vi "Drive.vi"(8 "error in":errorcluster) -> (0 "error out":errorcluster)   [LabVIEW 2016]
uses:
  Sprocket/src/Refname/Queues.ctl
  Sprocket/src/Refname/Actuators.ctl
  Drive States.ctl
  Sprocket/src/Action/Action Name.ctl
  Sprocket/src/Refname/Refname to String (Queue).vi
  <vilib>/addons/control/pid/pid.llb/PID (DBL).vi
  Main/Robot Global Data.vi
  Sprocket/lib/Sprocket.lvlib
  <vilib>/addons/control/pid/NI_PID_pid.lvlib
panel:
  in  "PID gains":T1={"proportional gain (Kc)"=0.025, "integral time (Ti, min)"=0.0, "derivative time (Td, min)"=0.0} {"derivative time (Td, min)" format="%.3f"; "integral time (Ti, min)" format="%.3f"; "proportional gain (Kc)" format="%.3f"}
  in  "output range":cluster{"output high":dbl, "output low":dbl}={"output high"=0.6, "output low"=-0.6} {"output low" format="%.2f"; "output high" format="%.2f"}
  # "Auto Rotate PID"
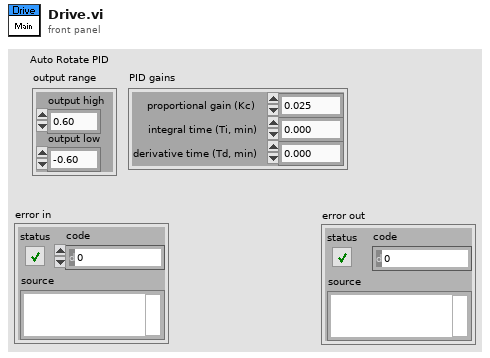
[diagram p1: front panel]
types:
  T1 = cluster{"proportional gain (Kc)":dbl, "integral time (Ti, min)":dbl, "derivative time (Td, min)":dbl}
  T2 = typedef "Sprocket.lvlib/Actuators.ctl" = enum16{"Drive Motor 1 (R)", "Drive Motor 2 (R)", "Drive Motor 3 (R)", "Drive Motor 4 (L)", "Drive Motor 5 (L)", "Drive Motor 6 (L)", "Collector Motor", "Collector Solenoid", "Compressor", "SonicShifter", "Gyro", "UltraSonic Front Left", "UltraSonic Back Left", "Wedge Motor", "Wedge LS"}
  T3 = typedef "Drive States.ctl" = enum16{"Idle", "Teleop", "Start Rotate", "Do Rotate", "Stop Rotate", "Start Throttle", "Do Throttle", "Stop Throttle"}
  T4 = typedef "Sprocket.lvlib/Queues.ctl" = enum16{"Input", "Drive", "Collector", "Shifter", "Wedge"}
  T5 = typedef "WPI_MotorControlDeviceRef.ctl" = cluster{"DeviceStatus":errorcluster, "Type":T6, "PWM":cluster{"PWM Channel":T7, "DeadBand":T8}, "CAN":cluster{"Device Number":u8, "SetOutput VI Ref":variant, "GetOutput VI Ref":variant, "Enable VI Ref":variant, "Disable VI Ref":variant, "Data":variant}, "Invert":bool}
  T6 = typedef "WPI_MotorControlType.ctl" = enum16{"PWM", "CAN"}
  T7 = typedef "FPGA_DIOPWMChannel.ctl" = enum8{"PWM 0", "PWM 1", "PWM 2", "PWM 3", "PWM 4", "PWM 5", "PWM 6", "PWM 7", "PWM 8", "PWM 9", "PWM MXP 0", "PWM MXP 1", "PWM MXP 2", "PWM MXP 3", "PWM MXP 4", "PWM MXP 5", "PWM MXP 6", "PWM MXP 7", "PWM MXP 8", "PWM MXP 9", "Invalid"}
  T8 = typedef "WPI_PWMDeadband.ctl" = cluster{"Name":string, "maxPositivePwm":i32, "minPositivePwm":i32, "centerPwm":i32, "maxNegativePwm":i32, "minNegativePwm":i32, "angularRange":u16}
  T9 = typedef "WPI_GyroDevRef.ctl" = cluster{"DevStatus":errorcluster, "Analog Channel":T10, "Offset":dbl, "Gain (VoltsPerDegree/Second)":dbl, "Gyro Type":enum16{"Analog", "XRS450"}, "Handle":i32, "SPI Bus":T11, "Device Found":bool, "Sample Rate":dbl, "Calibrate On Open":bool}
  T10 = typedef "FPGA_AIChannel.ctl" = enum8{"AI 0", "AI 1", "AI 2", "AI 3", "AI MXP 0", "AI MXP 1", "AI MXP 2", "AI MXP 3", "Invalid"}
  T11 = typedef "spi_bus.ctl" = enum16{"SPI On-Board, CS0", "SPI On-Board, CS1", "SPI On-Board, CS2", "SPI On-Board, CS3", "SPI MXP", "Invalid"}
  T12 = typedef "Sprocket.lvlib/Action Name.ctl" = enum16{"No Action", "Drive Train Both", "Drive Train Rotate", "Drive Train Throttle", "Collector Motor Roll", "Collector Motor Eject", "Collector Motor Collect", "Collector Motor Stop", "Collector Extend", "Collector Retract", "Shifter High", "Shifter Low", "Collector Motor Stall", "Wedge Roll"}
  T13 = typedef "Sprocket.lvlib/Action.ctl" = cluster{"Name":T12, "Priority":i32, "Data":variant}
  T14 = typedef "WPI_CANTalonSRX_GlobalStatus.ctl" = cluster{"Applied Throttle":dbl, "Module Enabled":bool, "CAN Error":errorcluster, "Closed Loop Error":dbl, "Forward Limit Switch Closed":bool, "Reverse Limit Switch Closed":bool, "Sensor Position":dbl, "Sensor Velocity":dbl, "Current":dbl, "Sticky Fault - Over Temp":bool, "Sticky Fault - Under Voltage":bool, "Sticky Fault - Forward Limit":bool, "Sticky Fault - Reverse Limit":bool, "Sticky Fault - Forward Soft Limit":bool, "Sticky Fault - Reverse Soft Limit":bool, "Brake is Enabled":bool, "Encoder Position":dbl, "Encoder Velocity":dbl, "Encoder Index Count":dbl, "Encoder A Pin State":bool, "Encoder B Pin State":bool, "Encoder Index Pin State":bool, "Analog In":dbl, "Analog In Velocity":dbl, "Temperature (C)":dbl, "Battery Voltage":dbl, "Control 5 Is Supported":bool, "Current Profile Slot Select":dbl, "Pos Div 8":bool, "Vel Div 4":bool, "Pulse Width Position":i32, "Pulse Width Velocity":i32, "Pulse Width Rise To Rise (us)":i32, "Pulse Width Rise To Fall (us)":i32, "Mot Prof Active Is Under Run":bool, "Mot Prof Active Has Under Run":bool, "Mot Prof Active Is Last":bool, "Mot Prof Active Velocity Only":bool, "Mot Prof Active Is Valid":bool, "Mot Prof Buffer Is Full":bool, "Mot Prof Active Profile Slot Select":i32, "Mot Prof NextID":i32, "Mot Prof Count":i32, "Mot Prof Active Velocity":dbl, "Mot Prof Active Position":dbl, "Mot Prof Output Enable":i32}
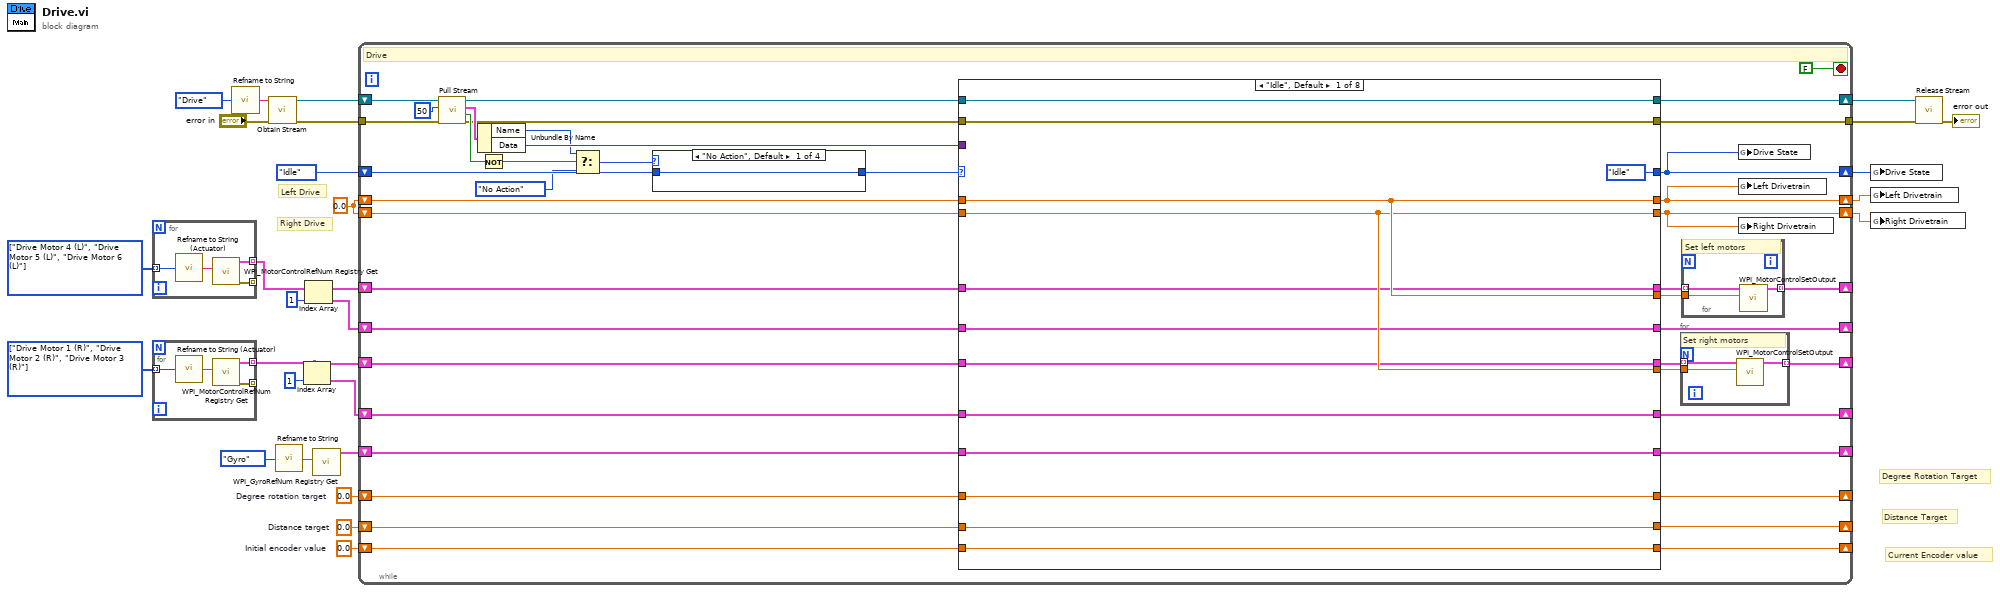
[diagram p0: block diagram]
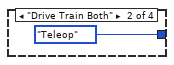
[diagram p2: hidden frame]
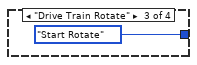
[diagram p3: hidden frame]
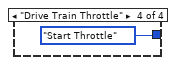
[diagram p4: hidden frame]
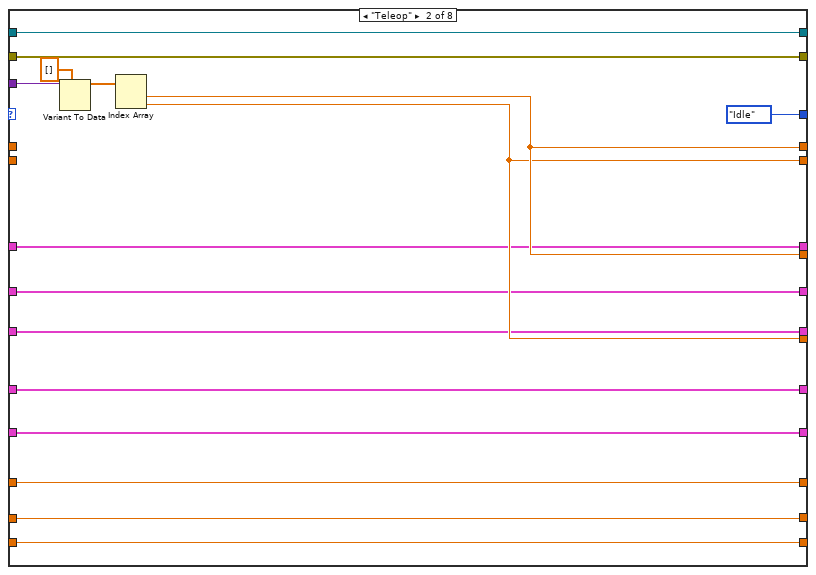
[diagram p5: hidden frame]
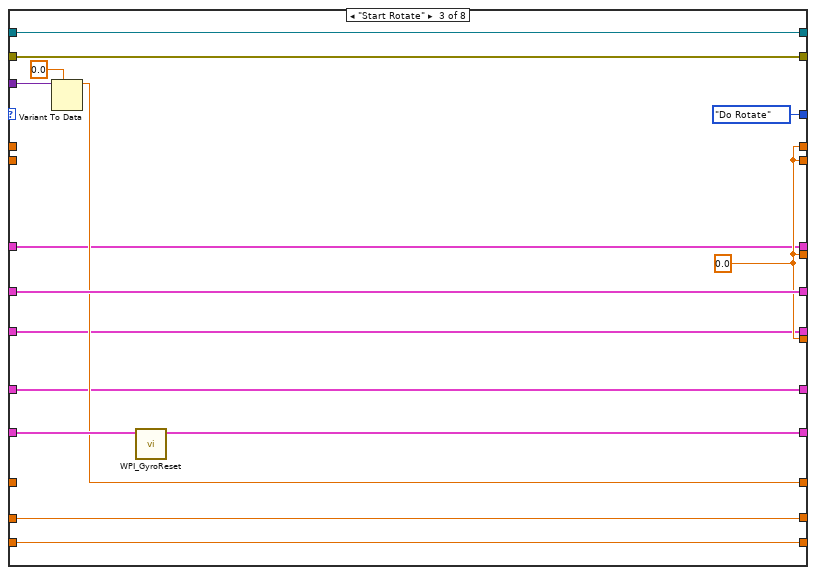
[diagram p6: hidden frame]
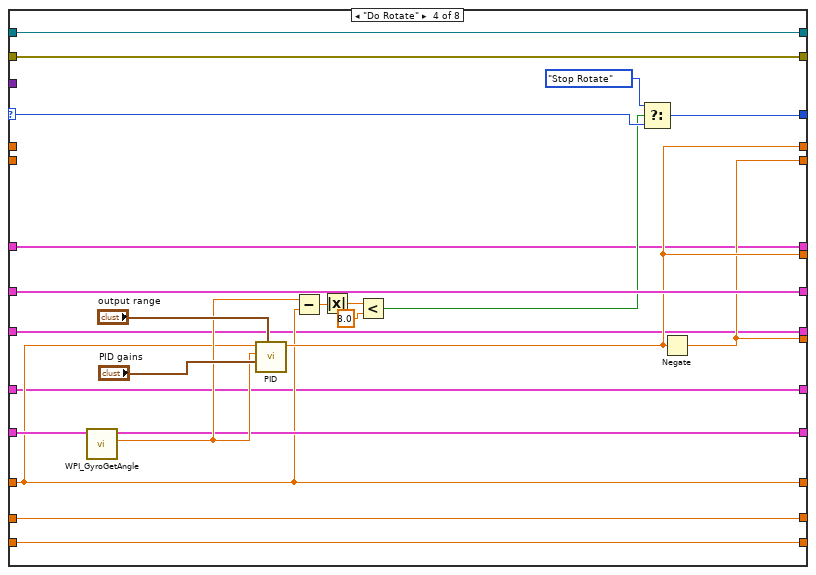
[diagram p7: hidden frame]
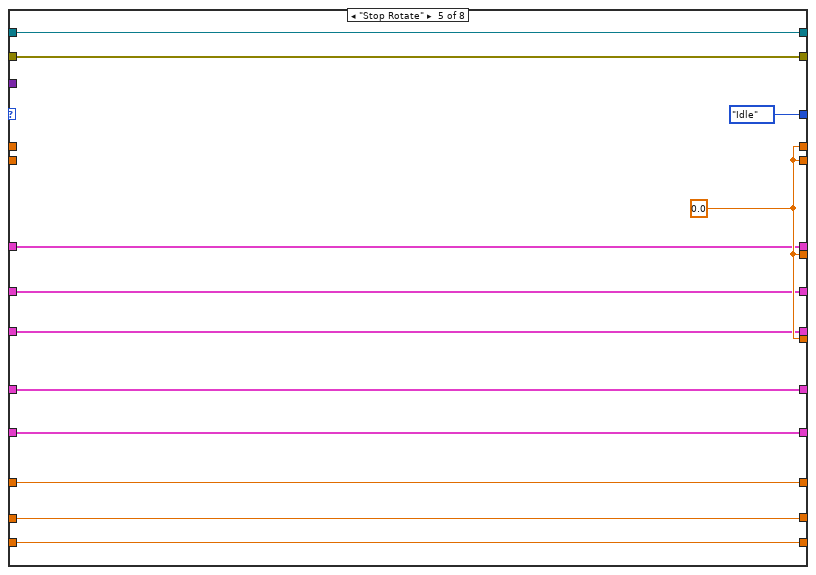
[diagram p8: hidden frame]
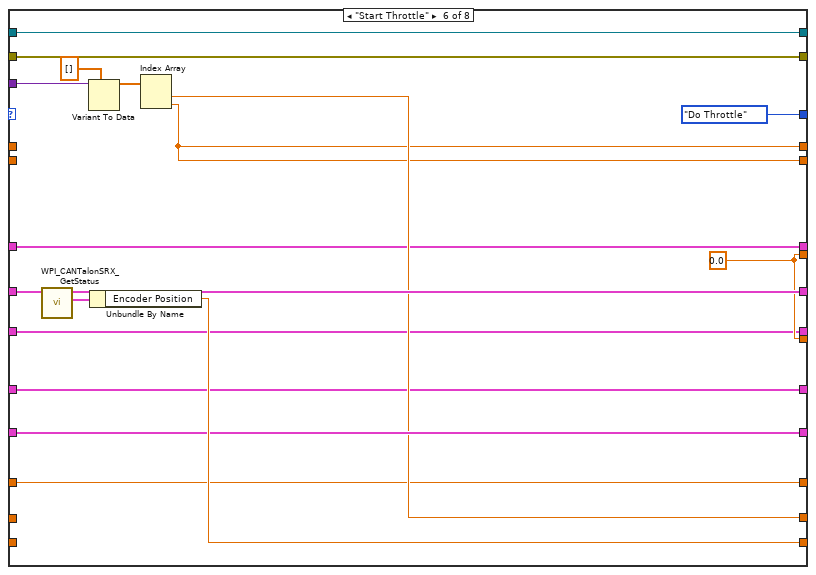
[diagram p9: hidden frame]
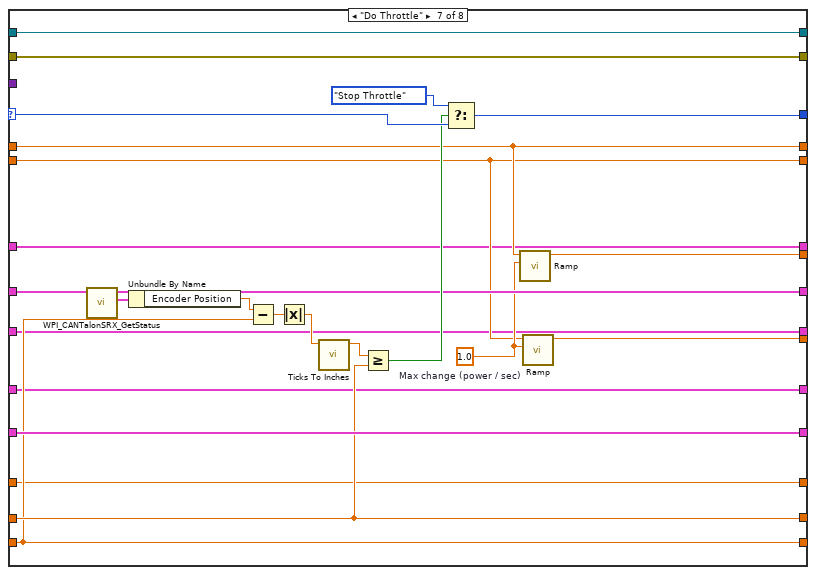
[diagram p10: hidden frame]
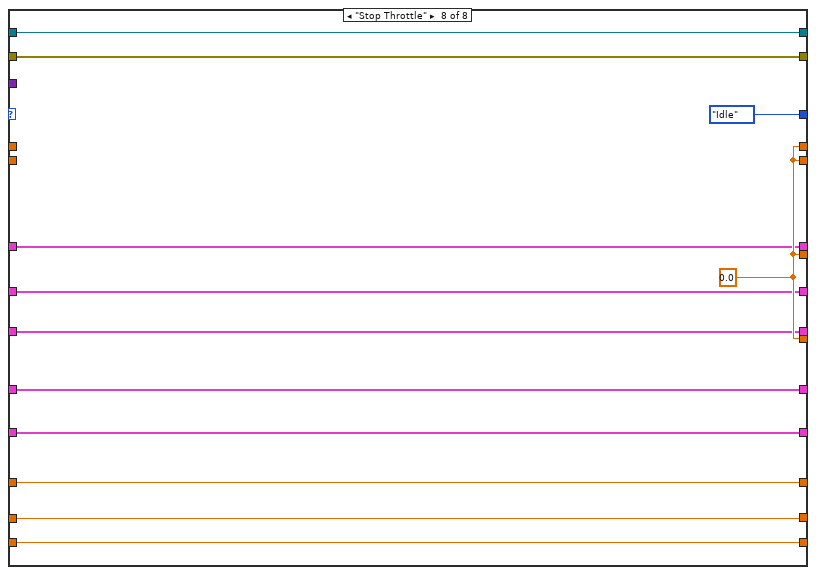
[diagram p11: hidden frame]
diagram:
  w5 = 0.0
  w15 = T2[] [enum."Drive Motor 4 (L)", enum."Drive Motor 5 (L)", enum."Drive Motor 6 (L)"] items=["Drive Motor 1 (R)", "Drive Motor 2 (R)", "Drive Motor 3 (R)", "Drive Motor 4 (L)", "Drive Motor 5 (L)", "Drive Motor 6 (L)", "Collector Motor", "Collector Solenoid", "Compressor", "SonicShifter", "Gyro", "UltraSonic Front Left", "UltraSonic Back Left", "Wedge Motor", "Wedge LS"]
  w17 = T2[] [enum."Drive Motor 1 (R)", enum."Drive Motor 2 (R)", enum."Drive Motor 3 (R)"] items=["Drive Motor 1 (R)", "Drive Motor 2 (R)", "Drive Motor 3 (R)", "Drive Motor 4 (L)", "Drive Motor 5 (L)", "Drive Motor 6 (L)", "Collector Motor", "Collector Solenoid", "Compressor", "SonicShifter", "Gyro", "UltraSonic Front Left", "UltraSonic Back Left", "Wedge Motor", "Wedge LS"]
  w20 = 0.0  # Initial encoder value
  w19 = 0.0  # Distance target
  w18 = 0.0  # Degree rotation target
  # "Right Drive"
  # "Left Drive"
  # "Current Encoder value"
  # "Distance Target"
  # "Degree Rotation Target"
  n1 = for {
    tunnel: w15 -> [w30] mode=indexing
    tunnel: [w29] -> _ mode=indexing
    tunnel: [w28] -> w10 mode=indexing
    n2 = call "Refname to String (Actuator).vi"("Actuator Refname"=w30) -> ("Refnum Name"=w31:string)
    n3 = call <vilib>:"WPI_MotorControlRefNum Registry Get.vi"("refnum name"=w31) -> ("error out"=w29:errorcluster, "MotorControlDevRef"=w28:T5)  [unwired: 9 in]
  }
  n4 = for {
    tunnel: w17 -> [w34] mode=indexing
    tunnel: [w33] -> _ mode=indexing
    tunnel: [w32] -> w1 mode=indexing
    n5 = call "Refname to String (Actuator).vi"("Actuator Refname"=w34) -> ("Refnum Name"=w35:string)
    n6 = call <vilib>:"WPI_MotorControlRefNum Registry Get.vi"("refnum name"=w35) -> ("error out"=w33:errorcluster, "MotorControlDevRef"=w32:T5)  [unwired: 9 in]
  }
  n7 = call-poly "Refname to String.vi"("Queue Refname"=Queues."Drive" ("Refname (Queue)")) -> ("Refnum Name"=w21:string)
  n8 = call "Obtain Stream.vi"("error in (no error)"="error in", "Name"=w21) -> ("error out"=w25:errorcluster, "stream out"=w24:refnum<queue>)  [unwired: 8 in]
  n9 = call-poly "Refname to String.vi"("Actuator Refname"=Actuators."Gyro") -> ("Refnum Name"=w13:string)
  n10 = Index Array(array=w1, index=1) -> (element=w2:T5)
  n11 = Index Array(array=w10, index=1) -> (element=w8:T5)
  n12 = call <vilib>:"WPI_GyroRefNum Registry Get.vi"("refnum name"=w13) -> ("GyroDevRef"=w11:T9)  [unwired: 9 in, 1 out]
  n13 = while {
    shift-right: [w45] -> w27
    shift-left: w24 -> [w72]
    shift-right: [w70] -> w3
    shift-left: w5 -> [w68]
    shift-right: [w71] -> w4
    shift-left: w5 -> [w69]
    tunnel: w25 -> [w73]
    tunnel: [w74] -> w26
    shift-right: [w58] -> _
    shift-left: w10 -> [w40]
    shift-right: [w57] -> _
    shift-left: w1 -> [w38]
    shift-right: [w62] -> _
    shift-left: w18 -> [w61]
    shift-right: [w54] -> _
    shift-left: w19 -> [w56]
    shift-right: [w53] -> _
    shift-left: w20 -> [w55]
    shift-right: [w51] -> w7
    shift-left: Drive_States."Idle" ("Enum") -> [w65]
    shift-right: [w63] -> _
    shift-left: w11 -> [w47]
    shift-right: [w52] -> _
    shift-left: w8 -> [w49]
    shift-right: [w36] -> _
    shift-left: w2 -> [w48]
    stop <- FALSE stop-if-true
    # "Drive"
    n14 = call "Pull Stream.vi"("error in (no error)"=w73, "timeout in ms (-1)"=50, "stream in"=w72) -> ("error out"=w41:errorcluster, "timed out?"=w67:bool, "element"=w76:T13, "queue out"=w46:refnum<queue>)  [unwired: 5 in]
    n15 = Unbundle By Name(w76) -> ("Name"=w43:T12, "Data"=w75:variant)
    n16 = Not(x=w67) -> (.not. x?=w44:bool)
    n17 = Select(t=w43, s=w44, f=Action_Name."No Action" ("Name")) -> (s? t:f=w66:T12)
    n18 = case shown="\"No Action\", Default" w66 {
      tunnel: [w84 Drive_States."Teleop" ("Enum") Drive_States."Start Rotate" ("Enum") Drive_States."Start Throttle" ("Enum")] -> w64
      tunnel: w65 -> [w84 _ _ _]
      frame "No Action", Default {
      }
      frame "Drive Train Both" {
      }
      frame "Drive Train Rotate" {
      }
      frame "Drive Train Throttle" {
      }
    }
    n19 = case shown="\"Idle\", Default" w64 {
      selector: w64 -> [_ _ _ w154 _ _ w205 _]
      tunnel: w75 -> [_ w116 w128 _ _ w184 _ _]
      tunnel: [w98 w111 w124 w142 w164 w175 w194 w220] -> w71
      tunnel: [w97 w110 w124 w141 w164 w175 w191 w220] -> w70
      tunnel: w68 -> [w97 _ _ _ _ _ w191 _]
      tunnel: w69 -> [w98 _ _ _ _ _ w194 _]
      tunnel: [w94 w101 w122 w132 w155 w171 w189 w216] -> w74
      tunnel: w47 -> [w99 w112 w131 w144 w165 w180 w199 w219]
      tunnel: [Drive_States."Idle" ("Enum") Drive_States."Idle" ("Enum") Drive_States."Do Rotate" ("Enum") w152 Drive_States."Idle" ("Enum") Drive_States."Do Throttle" ("Enum") w203 Drive_States."Idle" ("Enum")] -> w51
      tunnel: [w99 w112 w129 w140 w165 w180 w199 w219] -> w63
      tunnel: [w90 w104 w125 w139 w158 w170 w187 w212] -> w62
      tunnel: w61 -> [w90 w104 _ w139 w158 w170 w187 w212]
      tunnel: [w98 w111 w124 w142 w164 w174 w193 w220] -> w60
      tunnel: [w97 w110 w124 w141 w164 w174 w192 w220] -> w59
      tunnel: w56 -> [w89 w103 w121 w136 w157 _ w197 w211]
      tunnel: w55 -> [w88 w102 w120 w135 w156 _ w196 w210]
      tunnel: [w89 w103 w121 w136 w157 w176 w197 w211] -> w54
      tunnel: w49 -> [w96 w109 w127 w151 w163 w181 w202 w218]
      tunnel: [w88 w102 w120 w135 w156 w182 w196 w210] -> w53
      tunnel: [w96 w109 w127 w151 w163 w178 w198 w218] -> w52
      tunnel: w48 -> [w91 w105 w119 w134 w159 w167 w185 w213]
      tunnel: w46 -> [w95 w108 w123 w138 w162 w173 w190 w217]
      tunnel: [w95 w108 w123 w138 w162 w173 w190 w217] -> w45
      tunnel: w41 -> [w94 w101 w122 w132 w155 w171 w189 w216]
      tunnel: w40 -> [w93 w106 w117 w137 w161 w169 w188 w215]
      tunnel: [w93 w106 w117 w137 w161 w169 w188 w215] -> w39
      tunnel: w38 -> [w92 w107 w118 w133 w160 w168 w186 w214]
      tunnel: [w92 w107 w118 w133 w160 w168 w186 w214] -> w37
      tunnel: [w91 w105 w119 w134 w159 w167 w185 w213] -> w36
      frame "Idle", Default {
      }
      frame "Teleop" {
        n20 = Variant To Data(type=dbl[] [], Variant=w116) -> (data=w115:dbl[])  [unwired: 1 in, 1 out]
        n21 = Index Array(array=w115) -> (element #1=w111:dbl, element #2=w110:dbl)  [unwired: 2 in]
      }
      frame "Start Rotate" {
        w124 = 0.0
        n22 = Variant To Data(type=0.0, Variant=w128) -> (data=w125:dbl)  [unwired: 1 in, 1 out]
        n23 = call <vilib>:"WPI_GyroReset.vi"("GyroDevRef"=w131) -> ("GyroDevRef"=w129:T9)  [unwired: 9 in, 1 out]
      }
      frame "Do Rotate" {
        n24 = call <vilib>:"WPI_GyroGetAngle.vi"("GyroDevRef"=w144) -> ("Angle"=w145:dbl, "GyroDevRef"=w140:T9)  [unwired: 6 in, 3 out]
        n25 = call-poly <vilib>:"PID.vi"("output range"="output range", "PID gains"="PID gains", "process variable"=w145, "setpoint"=w139) -> ("output"=w142:dbl)  [unwired: 6 in, 1 out]
        n26 = Subtract(x=w145, y=w139) -> (x-y=w148:dbl)
        n27 = Absolute Value(x=w148) -> (abs(x)=w147:dbl)
        n28 = Less?(x=w147, y=8.0) -> (x < y?=w143:bool)
        n29 = Select(t=Drive_States."Stop Rotate", s=w143, f=w154) -> (s? t:f=w152:T3)
        n30 = Negate(x=w142) -> (-x=w141:dbl)
      }
      frame "Stop Rotate" {
        w164 = 0.0 ("Left Drive")
      }
      frame "Start Throttle" {
        w174 = 0.0 ("Left Drive")
        n31 = call <vilib>:"WPI_CANTalonSRX_GetStatus.vi"("CAN Talon SRX Ref"=w181) -> ("Talon SRX Status"=w183:T14, "CAN Talon SRX Ref"=w178:T5)  [unwired: 8 in, 1 out]
        n32 = Variant To Data(type=dbl[] [], Variant=w184) -> (data=w177:dbl[])  [unwired: 1 in, 1 out]
        n33 = Unbundle By Name(w183) -> ("Encoder Position"=w182:dbl)
        n34 = Index Array(array=w177) -> (element #1=w176:dbl, element #2=w175:dbl)  [unwired: 2 in]
      }
      frame "Do Throttle" {
        w195 = 1.0  # Max change (power / sec)
        n35 = call <vilib>:"WPI_CANTalonSRX_GetStatus.vi"("CAN Talon SRX Ref"=w202) -> ("Talon SRX Status"=w209:T14, "CAN Talon SRX Ref"=w198:T5)  [unwired: 8 in, 1 out]
        n36 = Unbundle By Name(w209) -> ("Encoder Position"=w200:dbl)
        n37 = Subtract(x=w200, y=w196) -> (x-y=w206:dbl)
        n38 = Absolute Value(x=w206) -> (abs(x)=w207:dbl)
        n39 = call "Ticks To Inches.vi"("Ticks"=w207) -> ("Inches"=w208:dbl)  [unwired: 9 in, 1 out]
        n40 = Greater Or Equal?(x=w208, y=w197) -> (x >= y?=w201:bool)
        n41 = Select(t=Drive_States."Stop Throttle" ("Enum"), s=w201, f=w205) -> (s? t:f=w203:T3)
        n42 = call "Ramp.vi"("Max change (power / sec)"=w195, "Joystick in"=w194) -> ("Motor out"=w193:dbl)  [unwired: 8 in, 1 out]
        n43 = call "Ramp.vi"("Max change (power / sec)"=w195, "Joystick in"=w191) -> ("Motor out"=w192:dbl)  [unwired: 8 in, 1 out]
      }
      frame "Stop Throttle" {
        w220 = 0.0
      }
    }
    n44 = for {
      tunnel: [w80] -> w57 mode=indexing
      tunnel: w59 -> [w79]
      tunnel: w37 -> [w78] mode=indexing
      # "Set right motors"
      n45 = call <vilib>:"WPI_MotorControlSetOutput.vi"("Output"=w79, "MotorControlDevRef"=w78) -> ("MotorControlDevRef"=w80:T5)  [unwired: 7 in, 2 out]
    }
    n46 = for {
      tunnel: [w83] -> w58 mode=indexing
      tunnel: w60 -> [w82]
      tunnel: w39 -> [w81] mode=indexing
      # "Set left motors"
      n47 = call <vilib>:"WPI_MotorControlSetOutput.vi"("Output"=w82, "MotorControlDevRef"=w81) -> ("MotorControlDevRef"=w83:T5)  [unwired: 7 in, 2 out]
    }
    n48 = global write "Robot Global Data.vi" "Drive State"(w51) -> ()
    n49 = global write "Robot Global Data.vi" "Left Drivetrain"(w71) -> ()
    n50 = global write "Robot Global Data.vi" "Right Drivetrain"(w70) -> ()
  }
  n51 = global write "Robot Global Data.vi" "Drive State"(w7) -> ()
  n52 = global write "Robot Global Data.vi" "Left Drivetrain"(w4) -> ()
  n53 = global write "Robot Global Data.vi" "Right Drivetrain"(w3) -> ()
  n54 = call "Release Stream.vi"("error in (no error)"=w26, "stream in"=w27) -> ("error out"=→"error out":errorcluster)  [unwired: 8 in, 1 out]
